vi "AB_Engine_RESTful_Get_ServiceVI_Info.vi"(8 "error in (no error)":errorcluster, 11 "sourceItems":refnum<class "AB_Source.lvclass">[](array[class])) -> (0 "error out":errorcluster, 1 "AuxVI paths":path[](array[path]), 2 "MethodVI  names":string[](array[string]), 3 "MethodVI paths":path[](array[path]), 5 "IncludedFile paths":path[](array[path]))   [LabVIEW 2020]
uses:
  <vilib>/AppBuilder/AB_Classes/Source/AB_Source.lvclass
  <vilib>/AppBuilder/AB_Classes/Source/RESTfulVI/AB_Source_RESTfulVI.lvclass
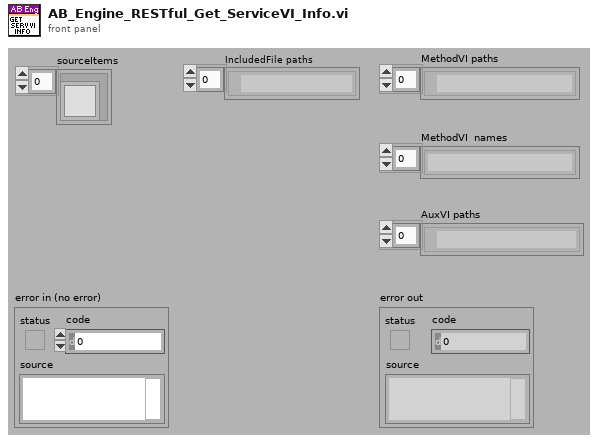
[diagram p1: front panel]
types:
  T1 = typedef "AB_Source.ctl" = cluster{"path":path, "itemID":string, "parentIndex":i32, "sourceInclusion":T2, "destinationIndex":i32, "properties":T3[], "newName":string, "lvfile":bool, "valid":bool, "eng_inBuild":bool, "eng_isNonVILink":bool, "Amalgamation":bool, "Amalgamation Piece":bool, "eng_delimitedName":string, "preventRename":bool}
  T2 = typedef "AB_Source_Inclusion.ctl" = enum16{"IncludeIfReferenced", "Include", "Exclude", "TopLevel"}
  T3 = typedef "AB_Source_Properties.ctl" = cluster{"sourcePropertyType":T4, "value":variant}
  T4 = typedef "AB_Source_Property_Type.ctl" = enum16{"Remove block diagram", "Remove front panel", "Password", "Window has title bar", "Show menu bar", "Show vertical scroll bar", "Show horizontal scroll bar", "Show toolbar", "Show Abort button", "Show fp when called", "Window behavior", "Allow user to close window", "Window run-time position", "Run when opened", "Allow debugging", "Auto error handling", "Generate guard code", "Use stack variables", "Expression folding", "Integer only", "Inline subVI"}
  T5 = typedef "AB_RESTful_Configuration.ctl" = cluster{"Service VI Type":T6, "Load VI at statup":bool, "Keep VI in memory":bool, "Output type":T7, "Output format":T8, "Use headers":bool, "Buffered":bool, "eng_Load VI by name":bool}
  T6 = typedef "AB_RESTful_VIType.ctl" = enum32{"Web Method", "Auxiliary", "eng_Internal", "eng_Content"}
  T7 = typedef "AB_RESTful_OutputType.ctl" = enum32{"Terminal", "Stream"}
  T8 = typedef "AB_RESTful_OutputFormat.ctl" = enum32{"XML", "Text", "HTML", "JSON"}
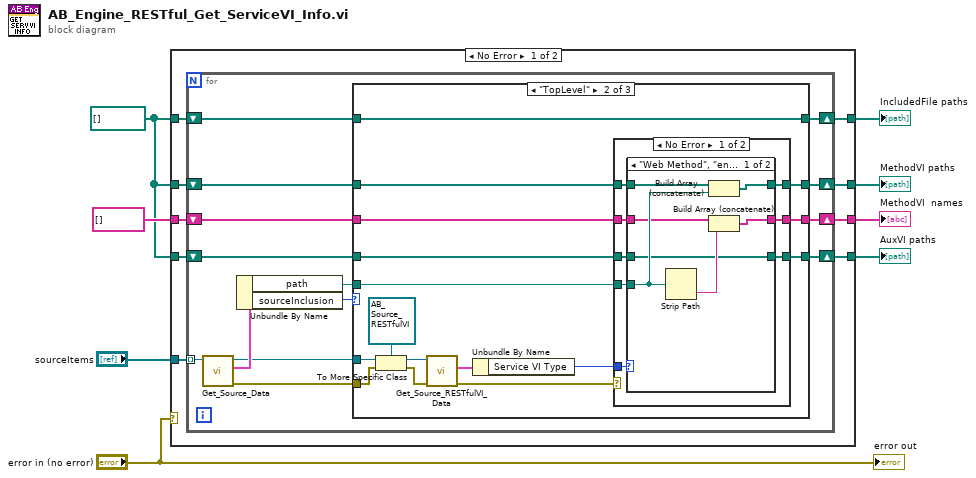
[diagram p0: block diagram]
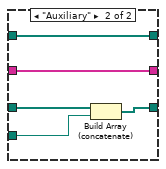
[diagram p3: hidden frame]
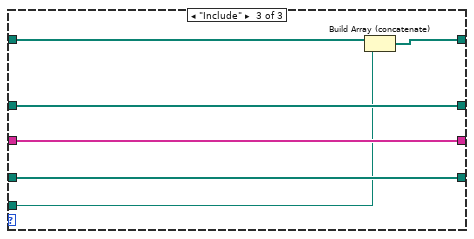
[diagram p5: hidden frame]
diagram:
  w2 = path[] []
  n1 = case shown="No Error" "error in (no error)" {
    tunnel: [w17 w84] -> w8
    tunnel: w2 -> [w16 w84]
    tunnel: "sourceItems" -> [w15 _]
    tunnel: string[] [] -> [w14 w83]
    tunnel: [w13 w83] -> w4
    tunnel: w2 -> [w12 w82]
    tunnel: [w11 w82] -> w3
    tunnel: w2 -> [w10 w81]
    tunnel: [w9 w81] -> w1
    frame No Error {
      n2 = for {
        tunnel: w15 -> [w30] mode=indexing
        shift-right: [w28] -> w17
        shift-left: w16 -> [w27]
        shift-right: [w23] -> w13
        shift-left: w14 -> [w22]
        shift-right: [w20] -> w11
        shift-left: w12 -> [w21]
        shift-right: [w18] -> w9
        shift-left: w10 -> [w19]
        n3 = call <vilib>:"Get_Source_Data.vi"("Class in"=w30) -> ("error out"=w24:errorcluster, "data"=w31:T1, "Class out"=w26:refnum<class "AB_Source.lvclass">)  [unwired: 8 in]
        n4 = Unbundle By Name(w31) -> ("path"=w29:path, "sourceInclusion"=w25:T2)
        n5 = case shown="\"TopLevel\"" w25 {
          tunnel: w29 -> [_ w51 w76]
          tunnel: [w35 w50 w80] -> w28
          tunnel: w27 -> [w35 w49 w80]
          tunnel: w26 -> [_ w48 _]
          tunnel: w24 -> [_ w43 _]
          tunnel: [w34 w42 w79] -> w23
          tunnel: w22 -> [w34 w41 w79]
          tunnel: w21 -> [w33 w38 w78]
          tunnel: [w33 w37 w78] -> w20
          tunnel: w19 -> [w32 w36 w77]
          tunnel: [w32 w36 w75] -> w18
          frame Default {
          }
          frame "TopLevel" {
            n6 = To More Specific Class(target class=refnum<class "AB_Source_RESTfulVI.lvclass"> refnum, reference=w48, error in=w43) -> (specific class reference=w46:refnum<class "AB_Source_RESTfulVI.lvclass">, error out=w45:errorcluster)
            n7 = call <vilib>:"Get_Source_RESTfulVI_Data.vi"("error in (no error)"=w45, "Class in"=w46) -> ("error out"=w40:errorcluster, "RESTful VI configuration"=w44:T5)  [unwired: 7 in, 1 out]
            n8 = Unbundle By Name(w44) -> ("Service VI Type"=w39:T6)
            n9 = case shown="No Error" w40 {
              tunnel: w51 -> [w57 _]
              tunnel: [w59 w74] -> w50
              tunnel: w49 -> [w58 w74]
              tunnel: [w56 w73] -> w42
              tunnel: w41 -> [w55 w73]
              tunnel: w39 -> [w54 _]
              tunnel: w38 -> [w53 w72]
              tunnel: [w52 w72] -> w37
              frame No Error {
                n10 = case shown="\"Web Method\", \"eng_Internal\", \"eng_Content\"" w54 {
                  tunnel: [w66 w71] -> w59
                  tunnel: w58 -> [w65 w71]
                  tunnel: w57 -> [w64 w69]
                  tunnel: [w62 w70] -> w56
                  tunnel: w55 -> [w61 w70]
                  tunnel: w53 -> [w60 w68]
                  tunnel: [w60 w67] -> w52
                  frame "Web Method", "eng_Internal", "eng_Content" {
                    n11 = Strip Path(path=w64) -> (name=w63:string)  [unwired: 1 out]
                    n12 = Build Array (concatenate)(w65, w64) -> (w66:path[])
                    n13 = Build Array (concatenate)(w61, w63) -> (w62:string[])
                  }
                  frame "Auxiliary" {
                    n14 = Build Array (concatenate)(w68, w69) -> (w67:path[])
                  }
                }
              }
              frame Error {
              }
            }
          }
          frame "Include" {
            n15 = Build Array (concatenate)(w77, w76) -> (w75:path[])
          }
        }
      }
    }
    frame Error {
    }
  }
  "MethodVI paths" <- w8
  "MethodVI  names" <- w4
  "AuxVI paths" <- w3
  "IncludedFile paths" <- w1
  "error out" <- "error in (no error)"
